vi "velScheduler.vi"(5 "max_v_sent":dbl=0.2 format="%#_13g", 6 "robotModel":dbl[][](array[numeric]), 7 "delta":dbl=0.2 format="%#_13g", 8 "error in (no error)":errorcluster, 9 "L":dbl=0.2 format="%#_13g", 10 "Dest_array in":T1(array[cluster]), 11 "Game in":refnum<class "Game.lvclass">) -> (0 "error out":errorcluster, 1 "backtracking_max_dest_vel_to_next_dest":dbl, 2 "Dest_array out":T1(array[cluster]), 3 "Game out":refnum<class "Game.lvclass">)   [LabVIEW 2023, in "Game.lvclass"]
uses:
  Game.lvclass
  <vilib>/Analysis/_algsub.llb/Real Vector Norm.vi
  <vilib>/Analysis/NI_AALPro.lvlib
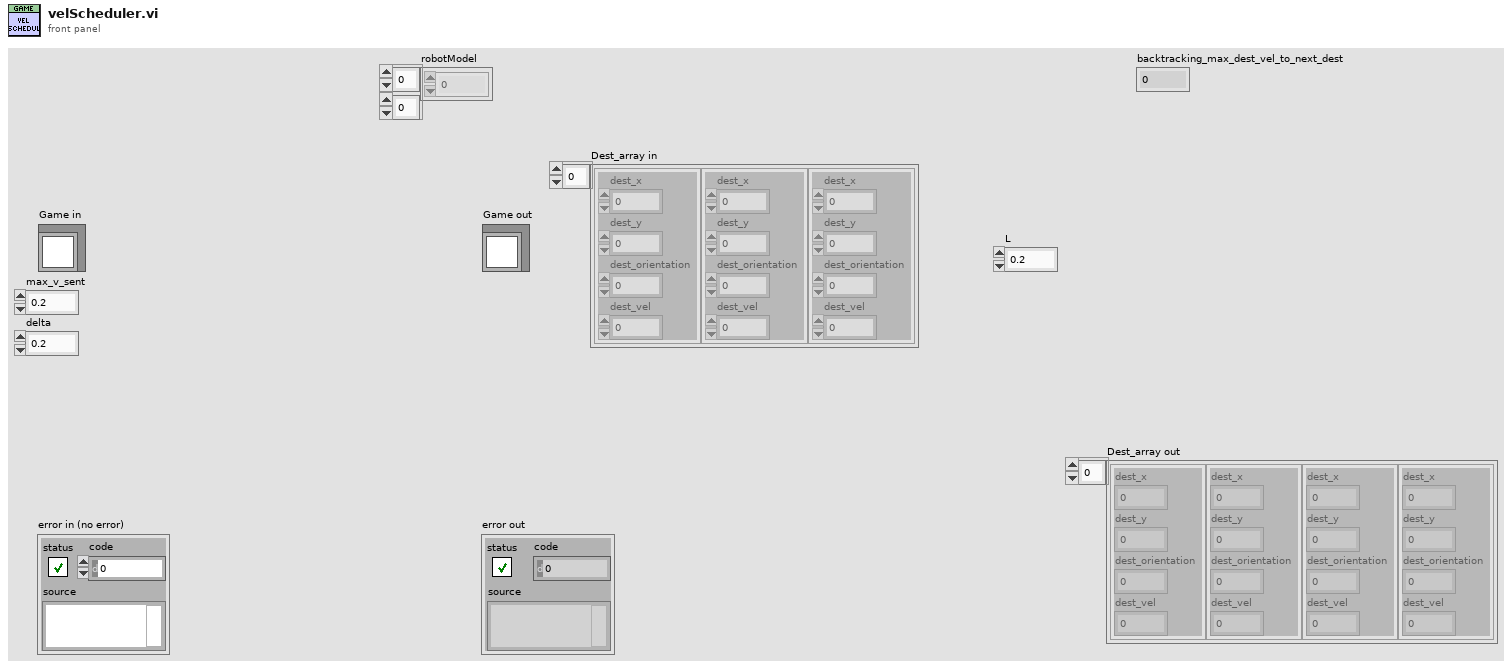
[diagram p1: front panel]
types:
  T1 = cluster{"dest_x":dbl, "dest_y":dbl, "dest_orientation":dbl, "dest_vel":dbl}[]
  T2 = cluster{"dest_x":dbl, "dest_y":dbl, "dest_orientation":dbl, "dest_vel":dbl}
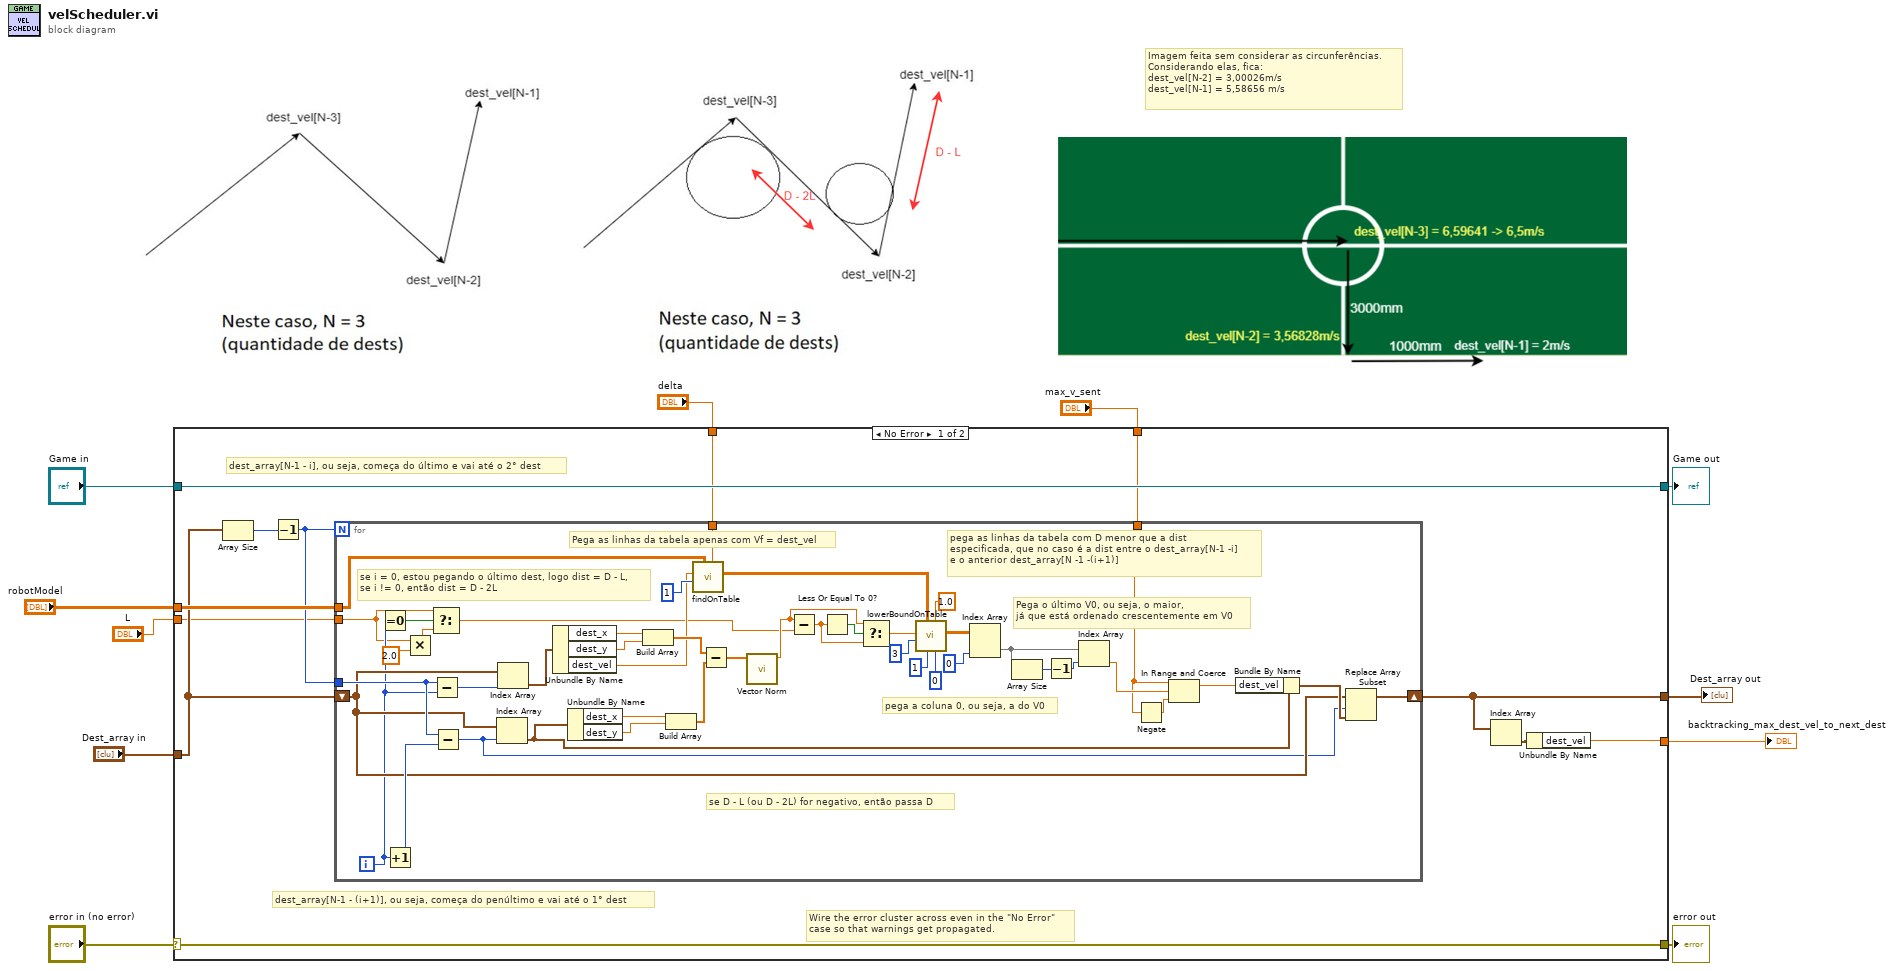
[diagram p0: block diagram]
diagram:
  # "Imagem feita sem considerar as circunferências.\nConsiderando elas, fica:\ndest_vel[N-2] = 3,00026m/s\ndest_vel[N-1] = 5,58656 m/s"
  n1 = case shown="No Error" "error in (no error)" {
    selector: "error in (no error)" -> [w22 w69]
    tunnel: [w22 w69] -> w10
    tunnel: [w23 w68] -> w8
    tunnel: "Game in" -> [w23 w68]
    tunnel: "robotModel" -> [w21 _]
    tunnel: "Dest_array in" -> [w16 _]
    tunnel: "max_v_sent" -> [w20 _]
    tunnel: "delta" -> [w19 _]
    tunnel: [w15 _] -> w5
    tunnel: [w13 _] -> w3
    tunnel: "L" -> [w12 _]
    frame No Error {
      # "dest_array[N-1 - (i+1)], ou seja, começa do penúltimo e vai até o 1° dest"
      # "dest_array[N-1 - i], ou seja, começa do último e vai até o 2° dest"
      # "Wire the error cluster across even in the \"No Error\"\ncase so that warnings get propagated."
      n2 = Array Size(array=w16) -> (size(s)=w18:i32)
      n3 = Decrement(x=w18) -> (x-1=w17:i32)
      n4 = for {
        N: w17 -> [_]
        tunnel: w21 -> [w67]
        tunnel: w20 -> [w48]
        tunnel: w19 -> [w47]
        tunnel: w17 -> [w45]
        shift-right: [w60] -> w15
        shift-left: w16 -> [w36]
        tunnel: w12 -> [w30]
        i -> [w33]
        # "se D - L (ou D - 2L) for negativo, então passa D"
        # "se i = 0, estou pegando o último dest, logo dist = D - L,\nse i != 0, então dist = D - 2L"
        # "Pega o último V0, ou seja, o maior,\njá que está ordenado crescentemente em V0"
        # "pega a coluna 0, ou seja, a do V0"
        # "pega as linhas da tabela com D menor que a dist\nespecificada, que no caso é a dist entre o dest_array[N-1 -i]\ne o anterior dest_array[N -1 -(i+1)]"
        # "Pega as linhas da tabela apenas com Vf = dest_vel"
        n5 = Equal To 0?(x=w33) -> (x = 0?=w32:bool)
        n6 = Increment(x=w33) -> (x+1=w44:i32)
        n7 = Multiply(x=w30, y=2.0) -> (x*y=w31:dbl)
        n8 = Select(t=w30, s=w32, f=w31) -> (s? t:f=w25:dbl)
        n9 = Subtract(x=w45, y=w33) -> (x-y=w46:i32)
        n10 = Subtract(x=w45, y=w44) -> (x-y=w35:i32)
        n11 = Index Array(array=w36, index=w35) -> (element=w39:T2)
        n12 = Index Array(array=w36, index=w46) -> (element=w40:T2)
        n13 = Unbundle By Name(w40) -> ("dest_x"=w43:dbl, "dest_y"=w42:dbl, "dest_vel"=w41:dbl)
        n14 = Unbundle By Name(w39) -> ("dest_x"=w38:dbl, "dest_y"=w37:dbl)
        n15 = Build Array(w43, w42) -> (w65:dbl[])
        n16 = Build Array(w38, w37) -> (w66:dbl[])
        n17 = call "findOnTable.vi"("delta"=w47, "table"=w67, "column"=1, "key"=w41) -> ("search_results"=w58:dbl[][])  [unwired: 5 in, 2 out]
        n18 = Subtract(x=w65, y=w66) -> (x-y=w64:dbl[])
        n19 = call-poly <vilib>:"Vector Norm.vi"("Input Vector"=w64) -> ("norm"=w26:dbl)  [unwired: 9 in, 1 out]
        n20 = Subtract(x=w26, y=w25) -> (x-y=w24:dbl)
        n21 = Less Or Equal To 0?(x=w24) -> (x <= 0?=w27:bool)
        n22 = Select(t=w26, s=w27, f=w24) -> (s? t:f=w28:dbl)
        n23 = call "lowerBoundOnTable.vi"("column_to_sort"=0, "sign"=1.0, "sign_idx"=1, "table"=w58, "target_idx"=3 ("column"), "key"=w28) -> ("search_results"=w59:dbl[][])  [unwired: 3 in, 2 out]
        n24 = Index Array(array=w59, index (col)=0 ("disabled index (col)")) -> (element=w54:dbl[])  [unwired: 1 in]
        n25 = Array Size(array=w54) -> (size(s)=w53:i32)
        n26 = Decrement(x=w53) -> (x-1=w52:i32)
        n27 = Index Array(array=w54, index=w52) -> (element=w51:dbl)
        n28 = Negate(x=w48) -> (-x=w49:dbl)
        n29 = In Range and Coerce(upper limit=w48, x=w51, lower limit=w49) -> (coerced(x)=w50:dbl)  [unwired: 1 out]
        n30 = Bundle By Name(cluster=w39, "dest_vel"=w50) -> (w61:T2)
        n31 = Replace Array Subset(array=w36, new element=w61, index=w35) -> (w60:T1)
      }
      n32 = Index Array(array=w15) -> (element=w14:T2)  [unwired: 1 in]
      n33 = Unbundle By Name(w14) -> ("dest_vel"=w13:dbl)
    }
    frame Error {
    }
  }
  "error out" <- w10
  "Game out" <- w8
  "Dest_array out" <- w5
  "backtracking_max_dest_vel_to_next_dest" <- w3
